vi "Analyze Data.vi"(8 "error in":errorcluster, 11 "CRDS in":refnum<class "CRDS.lvclass">) -> (0 "error out":errorcluster, 3 "CRDS out":refnum<class "CRDS.lvclass">)   [LabVIEW 2019, in "CRDS.lvclass"]
doc: "Analyze Data takes the stored ringdown data (1000 shots per cell) and:\n1) Calculates the ringdown decay constant tau\n2) Averages tau0 data as necessary\n3) Corrects the tau data for Rayleigh scattering\n4) Stores a 1-D array of taus returned on a 1 kHz basis (8k taus) if a jump drive (U:) is connected\n5) Flattens the data into a string and stuffs the string into the <b>data</b> shared variable for display on the UI.\n\nThis VI will not be called if the data is not \"good\" (that is, if an error was thrown in the <B>Get Data</B> routine. If an error is thrown while the data is being retrieved, then the data will not be sent to the UI."
uses:
  CRDS.lvclass
  CRDS.lvclass/CRDS.ctl
  Cell/CRDS Cell.lvclass/CRDS Cell.ctl
  Data/Main/Read filter.vi
  Data/Cell/CRDS Cell Data.lvclass
  Cell/CRDS Cell.lvclass
  Data/Main/CRDS Data.lvclass
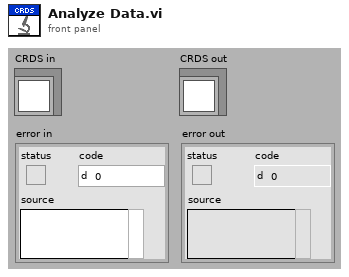
[diagram p1: front panel]
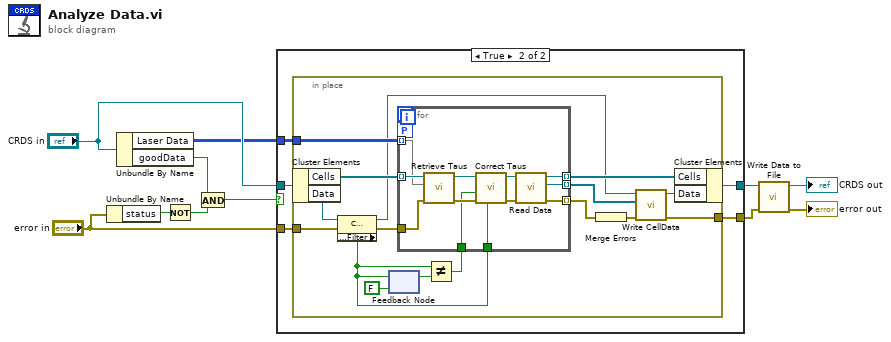
[diagram p0: block diagram]
diagram:
  n1 = Unbundle By Name("error in") -> ("status"=w9:bool)
  n2 = Unbundle By Name("CRDS in") -> ("Laser Data"=w7:i16[][][], "goodData"=w5:bool)
  n3 = Not(x=w9) -> (.not. x?=w8:bool)
  n4 = And(x=w5, y=w8) -> (x .and. y?=w6:bool)
  n5 = case shown="True" w6 {
    tunnel: "CRDS in" -> [w13 w16]
    tunnel: "error in" -> [w12 w18]
    tunnel: [w13 w15] -> w4
    tunnel: [w12 w14] -> w3
    tunnel: w7 -> [_ w17]
    frame False {
    }
    frame True {
      n6 = in-place {
        in-place-border: w18 -> [w28]
        in-place-border: [w25] -> w14
        in-place-border: w17 -> [w20]
        n7 = in-place-cluster #1(w16) -> ("Cells"=w24:refnum<class "CRDS Cell.lvclass">[], "Data"=w23:refnum<class "CRDS Data.lvclass">)
        n8 = property class="CRDS"(reference=w23, error in=w28) -> (reference out=w19:refnum<class "CRDS Data.lvclass">, error out=w27:errorcluster, "Data Access:Filter"=w29:bool)
        n9 = feedback #2(FALSE ("filter")) -> (w32:bool)
        n10 = feedback-in #2(w29) -> ()
        n11 = Not Equal?(x=w29, y=w32) -> (x != y?=w30:bool)
        n12 = for "Initial extinction calculation" {
          tunnel: w24 -> [w43] mode=indexing
          tunnel: w27 -> [w36]
          tunnel: w29 -> [w46]
          tunnel: [w40] -> w22 mode=indexing
          tunnel: [w39] -> w34 mode=indexing
          tunnel: [w38] -> w33 mode=indexing
          tunnel: w30 -> [w37]
          workers-P: _ -> [_]
          tunnel: w20 -> [w35] mode=indexing
          n13 = call "Retrieve Taus.vi"("error in"=w36, "Ringdowns"=w35, "CRDS Cell in"=w43) -> ("error out"=w44:errorcluster, "CRDS Cell out"=w45:refnum<class "CRDS Cell.lvclass">)  [unwired: 6 in, 1 out]
          n14 = call "Correct Taus.vi"("Filter?"=w46, "error in"=w44, "filter changed?"=w37, "CRDS Cell in"=w45) -> ("error out"=w41:errorcluster, "CRDS Cell out"=w42:refnum<class "CRDS Cell.lvclass">)  [unwired: 6 in]
          n15 = call "Read Data.vi"("error in"=w41, "CRDS Cell in"=w42) -> ("error out"=w39:errorcluster, "CRDS Cell"=w38:refnum<class "CRDS Cell Data.lvclass">, "CRDS Cell out"=w40:refnum<class "CRDS Cell.lvclass">)  [unwired: 7 in]
        }
        n16 = Merge Errors(w34) -> (w26:errorcluster)
        n17 = call "Write CellData.vi"("error in"=w26, "CellData"=w33, "CRDS Data in"=w19) -> ("error out"=w25:errorcluster, "CRDS Data out"=w21:refnum<class "CRDS Data.lvclass">)  [unwired: 7 in]
        n18 = in-place-cluster #1("Cells"=w22, "Data"=w21) -> (w15:refnum<class "CRDS.lvclass">)
      }
    }
  }
  n19 = call-dynamic "Write Data to File.vi"("error in (no error)"=w3, "Instrument in"=w4) -> ("error out"=→"error out":errorcluster, "Instrument out"=→"CRDS out":refnum<class "CRDS.lvclass">)  [unwired: 8 in]
